vi "Main.vi"() -> ()   [LabVIEW 2021]
doc: "The myRIO Project template acquires acceleration data from the onboard accelerometer and displays the changes of acceleration values in a waveform chart."
uses:
  <vilib>/userDefined/High Color/IMAQdx.ctl
  <vilib>/vision/driver/IMAQdx.llb/IMAQdx Camera Control Mode.ctl
  <vilib>/vision/driver/IMAQdx.llb/IMAQdx Acquisition Mode.ctl
  <vilib>/vision/driver/IMAQdx.llb/IMAQdx Buffer Number Mode.ctl
  <vilib>/vision/Management.llb/Cast Image 2 Method.ctl
  <vilib>/Platform/TimedLoop/XDataNode/timing_clust.ctl
  <vilib>/Platform/TimedLoop/XDataNode/nitl_modes.ctl
  <vilib>/Platform/TimedLoop/XDataNode/wakeup.ctl
  <vilib>/myRIO/Instrument Drivers/Onboard IO/DIO/typedefs/DIO Reference.ctl
  <vilib>/myRIO/Common/Instrument Driver Framework/Utilities/typedefs/myRIO Generic Hardware Reference.ctl
  <vilib>/myRIO/Common/Instrument Driver Framework/Utilities/typedefs/Hardware Version Enum.ctl
  <vilib>/myRIO/Common/Instrument Driver Framework/Utilities/typedefs/myRIO v1.0 Reference.ctl
  <vilib>/myRIO/Common/Instrument Driver Framework/Utilities/typedefs/Generic FPGA Reference.ctl
  <vilib>/myRIO/Common/Instrument Driver Framework/myRIO v1.0/DIO/typedefs/DIO Channels List.ctl
  <vilib>/myRIO/Common/Instrument Driver Framework/myRIO v1.0/DIO/typedefs/DIO Channels Enum.ctl
  <vilib>/userDefined/High Color/nirio_resource_hc.ctl
  <vilib>/myRIO/Instrument Drivers/Onboard IO/AI/typedefs/AI Reference.ctl
  <vilib>/myRIO/Common/Instrument Driver Framework/myRIO v1.0/AI/typedefs/AI Channels List.ctl
  <vilib>/myRIO/Common/Instrument Driver Framework/myRIO v1.0/AI/typedefs/AI Channels Enum.ctl
  <vilib>/myRIO/Common/Instrument Driver Framework/Utilities/typedefs/Analog Scaling Constants List.ctl
  <vilib>/myRIO/Common/Instrument Driver Framework/Utilities/typedefs/Analog Scaling Constants.ctl
  <vilib>/myRIO/Instrument Drivers/Onboard IO/PWM/typedefs/PWM Reference.ctl
  <vilib>/myRIO/Common/Instrument Driver Framework/myRIO v1.0/PWM/typedefs/PWM Channels Enum.ctl
  <vilib>/myRIO/Instrument Drivers/Onboard IO/PWM/typedefs/PWM Configuration.ctl
  <vilib>/myRIO/Common/Instrument Driver Framework/myRIO v1.0/DIO/vis/myRIO v1.1 Open DIO.vi
  <vilib>/myRIO/Common/Instrument Driver Framework/myRIO v1.0/AI/vis/myRIO v1.1 Open AI.vi
  <vilib>/myRIO/Common/Instrument Driver Framework/Utilities/vis/Is FPGA Ref Available.vi
  <vilib>/myRIO/Common/Instrument Driver Framework/myRIO v1.0/PWM/vis/myRIO v1.1 Open PWM.vi
  <vilib>/myRIO/Common/Instrument Driver Framework/Utilities/vis/Validate Channels.vi
  <vilib>/myRIO/Common/Instrument Driver Framework/myRIO v1.0/DIO/vis/myRIO v1.0 Reserve DIO.vi
  <vilib>/myRIO/Common/Instrument Driver Framework/myRIO v1.0/AI/vis/myRIO v1.0 Reserve AI.vi
  <vilib>/myRIO/Common/Instrument Driver Framework/myRIO v1.0/DIO/vis/myRIO v1.0 Close DIO.vi
  <vilib>/myRIO/Common/Instrument Driver Framework/myRIO v1.0/AI/vis/myRIO v1.0 Close AI.vi
  <vilib>/myRIO/Common/Instrument Driver Framework/myRIO v1.0/PWM/vis/myRIO v1.0 Reserve PWM.vi
  <vilib>/myRIO/Instrument Drivers/Onboard IO/PWM/vis/Set Duty Cycle and Frequency.vi
  <vilib>/myRIO/Common/Instrument Driver Framework/myRIO v1.0/PWM/vis/myRIO v1.0 Close PWM.vi
  <vilib>/myRIO/Common/Instrument Driver Framework/myRIO v1.0/Resource Manager/vis/myRIO v1.0 Reserve Channel List.vi
  <vilib>/myRIO/Common/Instrument Driver Framework/myRIO v1.0/DIO/vis/myRIO v1.0 Build MUX Configuration DIO.vi
  <vilib>/myRIO/Common/Instrument Driver Framework/myRIO v1.0/AI/vis/myRIO v1.0 Build MUX Configuration AI.vi
  <vilib>/myRIO/Common/Instrument Driver Framework/myRIO v1.0/DIO/vis/myRIO v1.0 Unreserve DIO.vi
  <vilib>/myRIO/Common/Instrument Driver Framework/myRIO v1.0/AI/vis/myRIO v1.0 Unreserve AI.vi
  <vilib>/myRIO/Common/Instrument Driver Framework/myRIO v1.0/PWM/vis/myRIO v1.0 Build MUX Configuration PWM.vi
  <vilib>/myRIO/Common/Instrument Driver Framework/myRIO v1.0/PWM/vis/myRIO v1.0 Unreserve PWM.vi
  <vilib>/myRIO/Common/Instrument Driver Framework/myRIO v1.0/Resource Manager/vis/myRIO v1.0 Reserve Channel.vi
  <vilib>/myRIO/Common/Instrument Driver Framework/myRIO v1.0/Resource Manager/vis/myRIO v1.0 Unreserve Channel.vi
  <vilib>/myRIO/Common/Instrument Driver Framework/myRIO v1.0/Resource Manager/vis/myRIO v1.0 Create Configuration List.vi
  <vilib>/myRIO/Common/Instrument Driver Framework/myRIO v1.0/Resource Manager/vis/myRIO v1.0 Unreserve Channel List.vi
  <vilib>/myRIO/Common/Instrument Driver Framework/myRIO v1.0/Resource Manager/vis/myRIO v1.0 Build Mutex Name.vi
  <vilib>/Utility/VariantDataType/GetNumericInfo.vi
  <vilib>/Utility/error.llb/Error Cluster From Error Code.vi
  <vilib>/myRIO/Common/Instrument Driver Framework/myRIO v1.0/myRIO v1.1 Open.vi
  <vilib>/myRIO/Common/Instrument Driver Framework/Utilities/vis/IO Manager.vi
  <vilib>/myRIO/Common/Instrument Driver Framework/Utilities/vis/Configuration Manager.vi
  <vilib>/myRIO/Common/Instrument Driver Framework/myRIO v1.0/Resource Manager/vis/myRIO v1.0 Configure IO.vi
  <vilib>/myRIO/Common/Instrument Driver Framework/myRIO v1.0/myRIO v1.0 Close.vi
  <vilib>/myRIO/Common/Instrument Driver Framework/myRIO v1.0/PWM/vis/myRIO v1.0 Write PWM.vi
  <vilib>/myRIO/Common/Instrument Driver Framework/myRIO v1.0/AI/vis/myRIO v1.0 Get Scaling Constants AI.vi
  <vilib>/myRIO/Common/Instrument Driver Framework/myRIO v1.0/DIO/vis/myRIO v1.0 Write DIO.vi
  <vilib>/myRIO/Common/Instrument Driver Framework/myRIO v1.0/AI/vis/myRIO v1.0 Read AI.vi
  <vilib>/myRIO/Common/Instrument Driver Framework/myRIO v1.0/DIO/vis/myRIO v1.0 Shutdown DIO.vi
  <vilib>/myRIO/Common/Instrument Driver Framework/myRIO v1.0/DIO/vis/myRIO v1.0 Read DIO.vi
  <vilib>/myRIO/Common/Instrument Driver Framework/myRIO v1.0/PWM/vis/myRIO v1.0 Shutdown PWM.vi
  <vilib>/myRIO/Instrument Drivers/Onboard IO/PWM/vis/myRIO PWM Open.xnode
  <vilib>/myRIO/Instrument Drivers/Onboard IO/AI/vis/myRIO AI Open.xnode
  <vilib>/myRIO/Instrument Drivers/Onboard IO/DIO/vis/myRIO DIO Open.xnode
  <vilib>/platform/TimedLoop/XDataNode/XDataNode.xnode
  <vilib>/myRIO/Express VI/Onboard Devices/LED/LED Express VI.xnode
  <vilib>/vision/driver/NI_Vision_Acquisition_Software.lvlib
  <vilib>/vision/NI_Vision_Development_Module.lvlib
  <vilib>/myRIO/Instrument Drivers/Onboard IO/PWM/PWM.lvlib
  <vilib>/myRIO/Instrument Drivers/Onboard IO/DIO/DIO.lvlib
  <vilib>/myRIO/Instrument Drivers/Onboard IO/AI/AI.lvlib
  <vilib>/Platform/TimedLoop/XDataNode/XDNodeRunTimeDep.lvlib
panel:
  in  "error in (no error) 3":errorcluster
  out "Darkness level":dbl(slide) scale=0.0..1.0
  out "Numeric":dbl format="%.2f"
  in  "error in (no error) 2":errorcluster
  in  "error in (no error)":errorcluster
  out "error out 2":errorcluster
  out "error out":errorcluster
  in  "Stop":bool
  out "Image":T1(plugin-control)
  out "Is Colour from Sample Detected":bool
  out "Number of Circles Returned":i32
  out "Match Score":i32[](array[numeric])
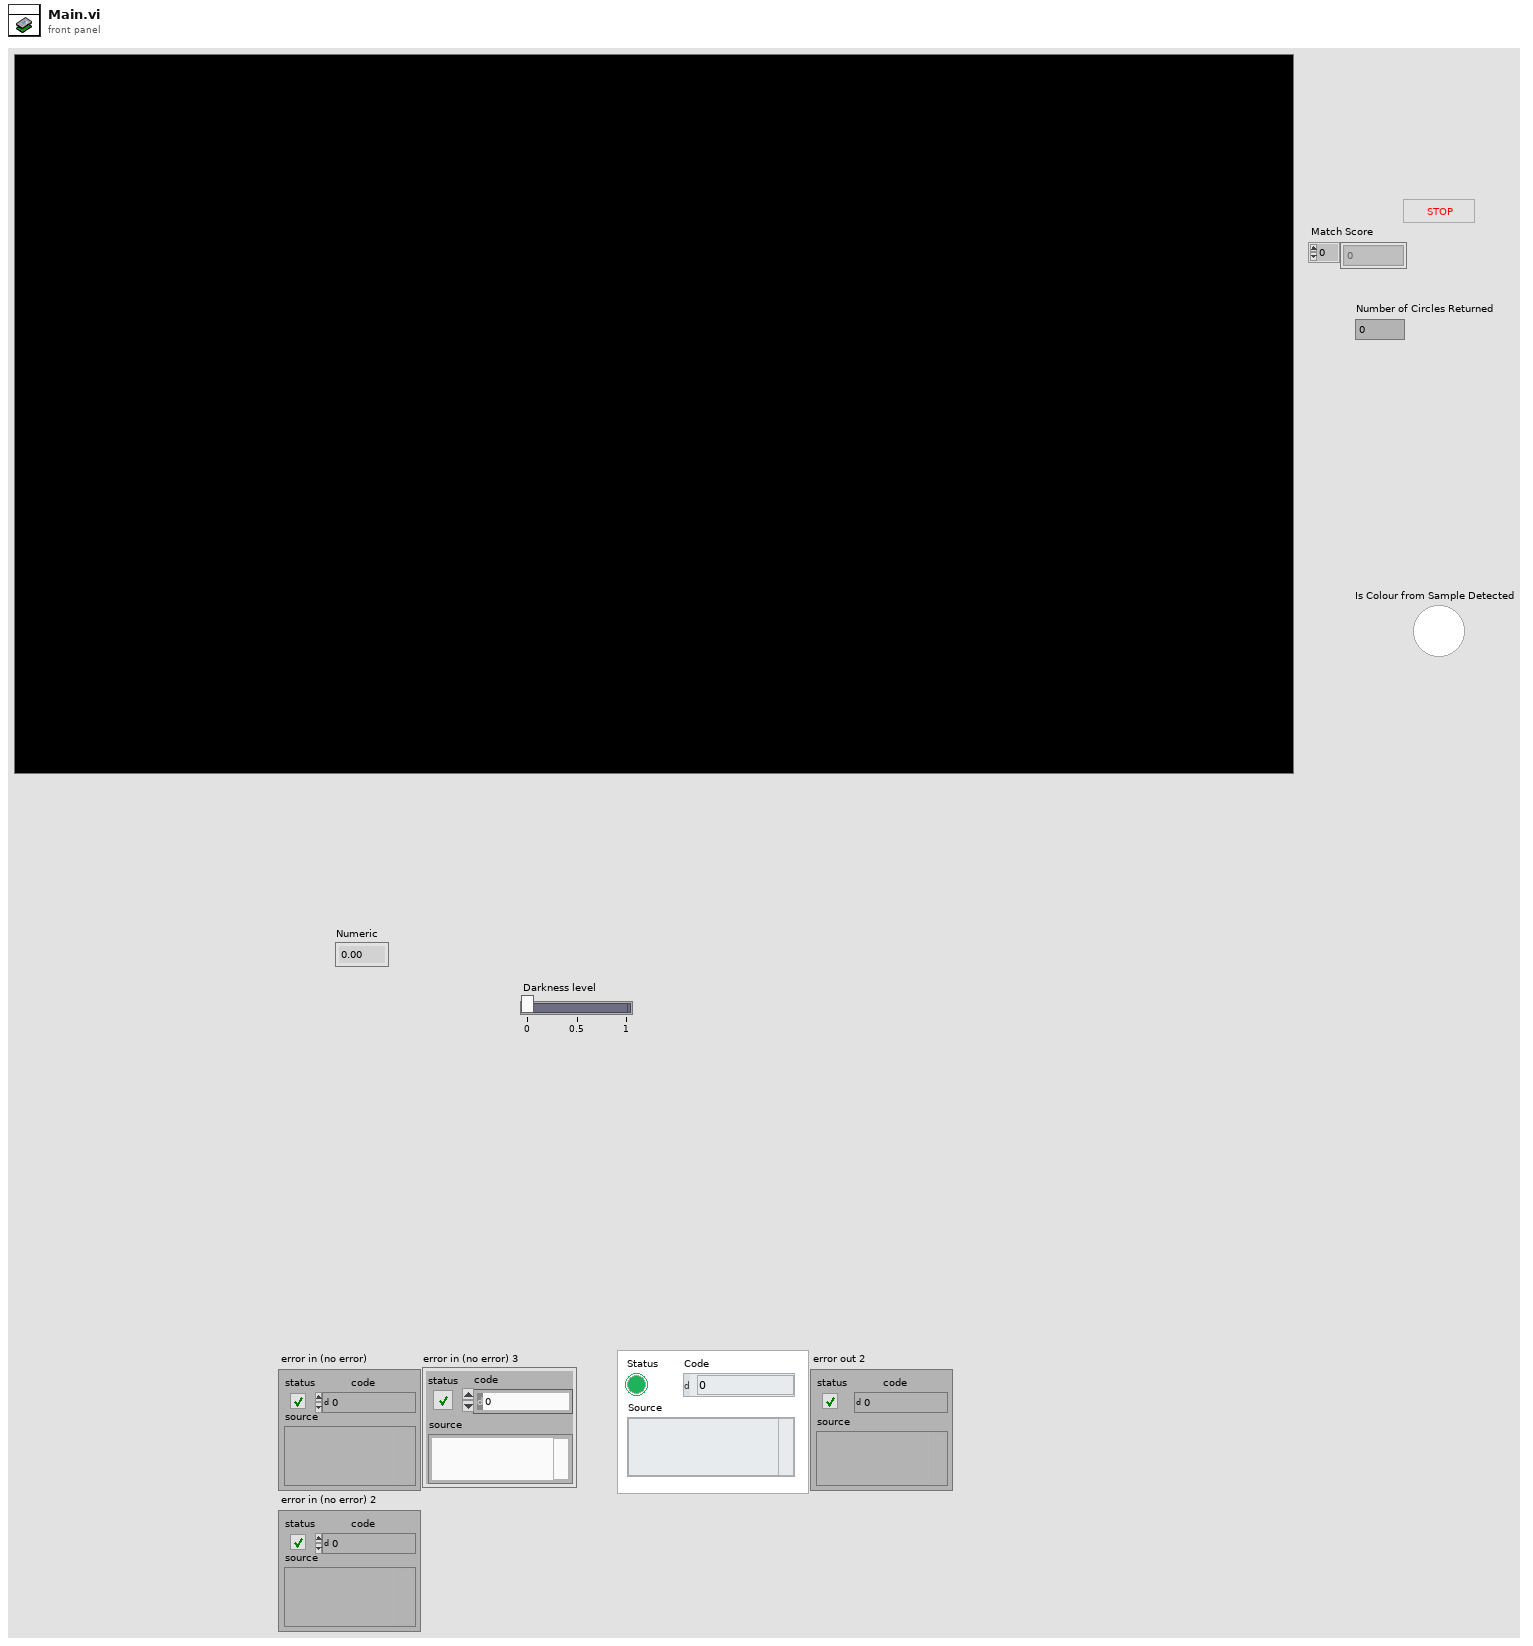
[diagram p1: front panel]
types:
  T1 = typedef "IMAQ Image.ctl" = refnum<image>
  T2 = typedef "Image Type" = u32
  T3 = typedef "Cast Image 2 Method.ctl" = u32
  T4 = typedef "IMAQ Rectangle" = cluster{"Left":i32, "Top":i32, "Right":i32, "Bottom":i32, "Rotation":dbl}
  T5 = typedef "NI_Vision_Acquisition_Software.lvlib/IMAQdx Buffer Number Mode.ctl" = enum32{"Next", "Last", "Buffer Number", "Every", "Last New"}
  T6 = typedef "NI_Vision_Acquisition_Software.lvlib/IMAQdx Acquisition Mode.ctl" = enum32{"One Shot", "Continuous"}
  T7 = typedef "NI_Vision_Acquisition_Software.lvlib/IMAQdx Camera Control Mode.ctl" = enum32{"Controller", "Listener"}
  T8 = typedef "IMAQdx.ctl" = refnum<k21>
  T9 = typedef "DIO.lvlib/DIO Reference.ctl" = cluster{"myRIO Reference":T10, "DIO Channels List":T14}
  T10 = typedef "myRIO Generic Hardware Reference.ctl" = cluster{"myRIO Model":T11, "myRIO Hardware Reference":T12}
  T11 = typedef "Hardware Version Enum.ctl" = enum16{"Unknown", "myRIO-1900", "myRIO-1950", "roboRIO", "NI ELVIS RIO CM", "ELVIS III"}
  T12 = typedef "myRIO v1.0 Reference.ctl" = cluster{"Generic FPGA Reference":T13, "Allow multiple opens":bool}
  T13 = typedef "Generic FPGA Reference.ctl" = refnum<k20>
  T14 = typedef "DIO Channels List.ctl" = T15[]
  T15 = typedef "DIO Channels Enum.ctl" = enum16{"Not Connected", "C/DIO0", "C/DIO1", "C/DIO2", "C/DIO3", "C/DIO4", "C/DIO5", "C/DIO6", "C/DIO7", "A/DIO0", "A/DIO1", "A/DIO2", "A/DIO3", "A/DIO4", "A/DIO5", "A/DIO6", "A/DIO7", "A/DIO8", "A/DIO9", "A/DIO10", "A/DIO11", "A/DIO12", "A/DIO13", "A/DIO14", "A/DIO15", "A/DIO16", "A/DIO17", "A/DIO18", "A/DIO19", "B/DIO0", "B/DIO1", "B/DIO2", "B/DIO3", "B/DIO4", "B/DIO5", "B/DIO6", "B/DIO7", "B/DIO8", "B/DIO9", "B/DIO10", "B/DIO11", "B/DIO12", "B/DIO13", "B/DIO14", "B/DIO15", "B/DIO16", "B/DIO17", "B/DIO18", "B/DIO19", "LED0", "LED1", "LED2", "LED3", "Button0", "DIO/DIO0", "DIO/DIO1", "DIO/DIO2", "DIO/DIO3", "DIO/DIO4", "DIO/DIO5", "DIO/DIO6", "DIO/DIO7", "DIO/DIO8", "DIO/DIO9", "SPI/CS0", "SPI/CS1", "SPI/CS2", "SPI/CS3", "LED RADIO (Green)", "LED RADIO (Red)", "LED COMM (Green)", "LED COMM (Red)", "LED MODE (Green)", "LED MODE (Red)"}
  T16 = typedef "XDNodeRunTimeDep.lvlib/timing_clust.ctl" = cluster{"Expected End [f-1]":u64, "Actual End [f-1]":u64, "Finished Late? [f-1]":bool, "Expected End [i-1]":u64, "Actual End [i-1]":u64, "Finished Late? [i-1]":bool, "Expected Start [i]":u64, "Actual Start [i]":u64, "Expected Start [f]":u64, "Actual Start [f]":u64, "Source Name":string, "Structure Name":string, "Period":i64, "Deadline":i64, "Offset":i64, "Start":i64, "Priority":i32, "Timeout":i32, "Mode":T17, "Wakeup Reason":T18, "Error":errorcluster, "Source Type":string, "Secondary Source Type":string, "Global End Time":u64, "Global Start Time":u64, "Frame Duration":u64, "Iteration Duration":u64, "Assigned CPU":i32, "I/O Scan Engine Mode":u32}
  T17 = typedef "XDNodeRunTimeDep.lvlib/nitl_modes.ctl" = enum32{"No Change", "Process missed periods, maintain original phase", "Discard missed periods, maintain original phase", "Process missed periods, ignore original phase", "Discard missed periods, ignore original phase"}
  T18 = typedef "XDNodeRunTimeDep.lvlib/wakeup.ctl" = enum32{"Normal", "Aborted", "Asynchronous wakeup", "Timing source error", "Timed loop error", "Timeout"}
  T19 = typedef "AI.lvlib/AI Reference.ctl" = cluster{"myRIO Reference":T10, "AI Channels List":T20, "AI Scaling Constants List":T22}
  T20 = typedef "AI Channels List.ctl" = T21[]
  T21 = typedef "AI Channels Enum.ctl" = enum16{"Not Connected", "AudioIn/Left", "AudioIn/Right", "C/AI0", "C/AI1", "A/AI0", "A/AI1", "A/AI2", "A/AI3", "A/AI4", "A/AI5", "A/AI6", "A/AI7", "B/AI0", "B/AI1", "B/AI2", "B/AI3", "B/AI4", "B/AI5", "B/AI6", "B/AI7", "AI/AI0", "AI/AI1", "AI/AI2", "AI/AI3", "A/AI0 (DIFF)", "A/AI1 (DIFF)", "A/AI2 (DIFF)", "A/AI3 (DIFF)", "B/AI0 (DIFF)", "B/AI1 (DIFF)", "B/AI2 (DIFF)", "B/AI3 (DIFF)"}
  T22 = typedef "Analog Scaling Constants List.ctl" = T23[]
  T23 = typedef "Analog Scaling Constants.ctl" = cluster{"LSB Weight (Volts)":dbl, "Offset (Volts)":dbl, "Signed?":bool}
  T24 = typedef "nirio_resource_hc.ctl" = tag
  T25 = typedef "PWM.lvlib/PWM Reference.ctl" = cluster{"myRIO Reference":T10, "PWM Channels Enum":T26, "PWM Configuration":T27}
  T26 = typedef "PWM Channels Enum.ctl" = enum16{"Not Connected", "C/PWM0", "C/PWM1", "A/PWM0", "A/PWM1", "A/PWM2", "A/PWM3", "A/PWM4", "A/PWM5", "A/PWM6", "A/PWM7", "A/PWM8", "A/PWM9", "A/PWM10", "A/PWM11", "A/PWM12", "A/PWM13", "A/PWM14", "A/PWM15", "A/PWM16", "A/PWM17", "A/PWM18", "A/PWM19", "B/PWM0", "B/PWM1", "B/PWM2", "B/PWM3", "B/PWM4", "B/PWM5", "B/PWM6", "B/PWM7", "B/PWM8", "B/PWM9", "B/PWM10", "B/PWM11", "B/PWM12", "B/PWM13", "B/PWM14", "B/PWM15", "B/PWM16", "B/PWM17", "B/PWM18", "B/PWM19", "PWM/PWM0", "PWM/PWM1", "PWM/PWM2", "PWM/PWM3", "PWM/PWM4", "PWM/PWM5", "PWM/PWM6", "PWM/PWM7", "PWM/PWM8", "PWM/PWM9"}
  T27 = typedef "PWM.lvlib/PWM Configuration.ctl" = cluster{"Frequency":dbl, "Duty Cycle":dbl}
  T28 = typedef "ROI Descriptor" = cluster{"Global Rectangle":i32[], "Contours":cluster{"ID":enum32{"External", "Internal"}, "Type":u32, "Coordinates":i32[]}[]}
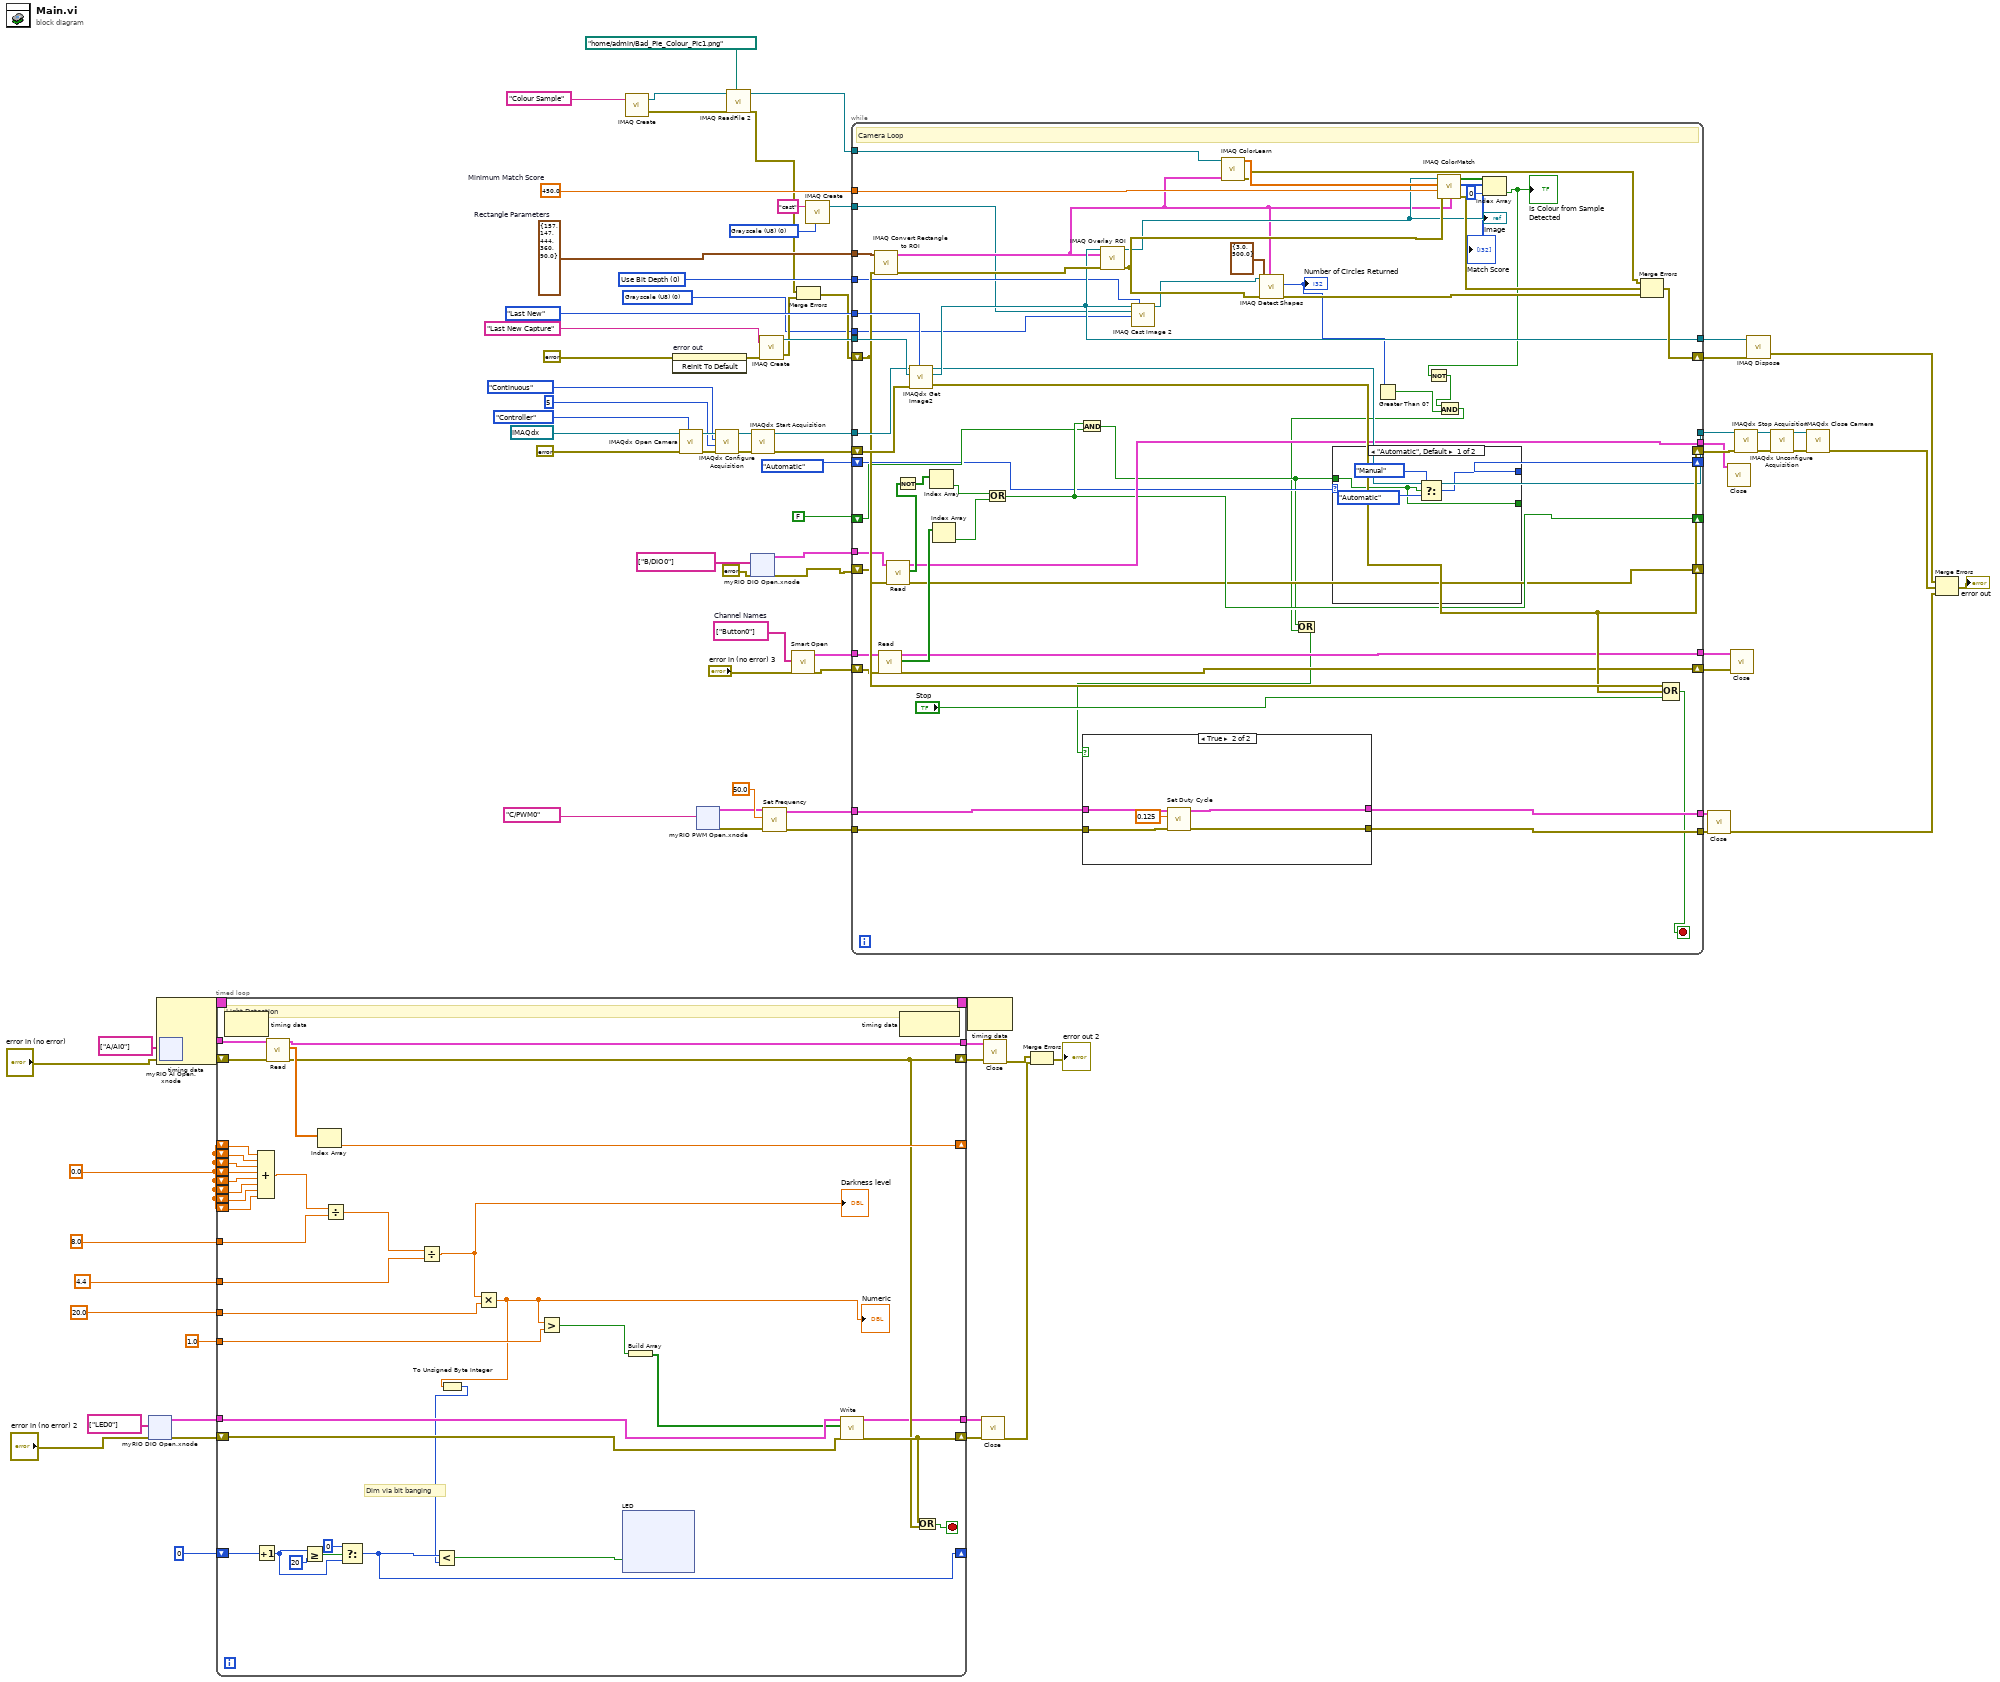
[diagram p0: block diagram]
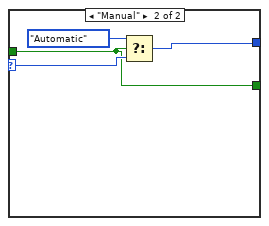
[diagram p2: hidden frame]
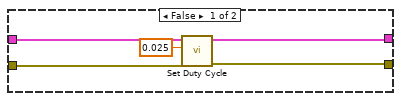
[diagram p3: hidden frame]
diagram:
  w12 = tag[] ["Button0"]  # Channel Names
  w30 = 0.0
  w36 = T2 0 items=["Grayscale (U8)", "Grayscale (I16)", "Grayscale (SGL)", "Complex (CSG)", "RGB (U32)", "HSL (U32)", "RGB (U64)", "Grayscale (U16)"] ("Image Type")
  w42 = T3 0 items=["Use Bit Depth", "Shift", "Use Lookup Table"] ("Method")
  w43 = T2 0 items=["Grayscale (U8)", "Grayscale (I16)", "Grayscale (SGL)", "Complex (CSG)", "RGB (U32)", "HSL (U32)", "RGB (U64)", "Grayscale (U16)"] ("Image Type")
  w53 = 450.0  # Minimum Match Score
  w60 = T4 {"Left"=157, "Top"=147, "Right"=444, "Bottom"=360, "Rotation"=90.0}  # Rectangle Parameters
  n1 = xnode "myRIO DIO Open.xnode"("error in (no error)"="error in (no error) 2", "Channel Names"=tag[] ["LED0"]) -> ("error out"=w25:errorcluster, "DIO Ref Out"=w26:T9)  [unwired: 1 in]
  n2 = node-c288() -> (w87:T16)  [unwired: 4 in]
  n3 = xnode "myRIO AI Open.xnode"("error in (no error)"="error in (no error)", "Channel Names"=tag[] ["A/AI0"]) -> ("error out"=w33:errorcluster, "AI Ref Out"=w34:T19)  [unwired: 1 in]
  n4 = timed-loop {
    tunnel: w34 -> [w124]
    shift-right: [w102] -> w32
    shift-left: w33 -> [w123]
    tunnel: [w122] -> w31
    shift-right: [w112] -> _
    shift-left: w30 -> [w114]
    shift-left: w30 -> [w115]
    shift-left: w30 -> [w116]
    shift-left: w30 -> [w117]
    shift-left: w30 -> [w118]
    shift-left: w30 -> [w119]
    shift-left: w30 -> [w120]
    shift-left: w30 -> [w121]
    tunnel: 8.0 -> [w111]
    tunnel: 4.4 -> [w109]
    tunnel: 20.0 -> [w107]
    tunnel: w26 -> [w105]
    shift-right: [w103] -> w24
    shift-left: w25 -> [w104]
    tunnel: [w101] -> w23
    tunnel: 1.0 ("y") -> [w99]
    shift-right: [w91] -> _
    shift-left: u8 0 -> [w93]
    timing: w87 -> [_]
    timing-out: [_] -> w86
    stop <- w100 stop-if-true
    # "Dim via bit banging"
    # "Light Detection"
    n5 = node-c288() -> ()  [unwired: 1 in, 1 out]
    n6 = Increment(x=w93) -> (x+1=w88:u8)
    n7 = Compound Arithmetic op=ADD(w114, w115, w116, w117, w118, w119, w120, w121) -> (w110:dbl)
    n8 = call <vilib>:"Read.vi"("error in (no error)"=w123, "AI Ref In"=w124) -> ("error out"=w102:errorcluster, "Values"=w113:dbl[], "AI Ref Out"=w122:T19)  [unwired: 7 in]
    n9 = Greater Or Equal?(x=w88, y=u8 20) -> (x >= y?=w95:bool)
    n10 = Index Array(array=w113) -> (element=w112:dbl)  [unwired: 1 in]
    n11 = Divide(x=w110, y=w111) -> (x/y=w108:dbl)
    n12 = Select(t=u8 0, s=w95, f=w88) -> (s? t:f=w91:u8)
    n13 = Divide(x=w108, y=w109) -> (x/y=w106:dbl)
    "Darkness level" <- w106
    n14 = Multiply(x=w106, y=w107) -> (x*y=w90:dbl)
    "Numeric" <- w90
    n15 = To Unsigned Byte Integer(number=w90) -> (unsigned 8bit integer=w89:u8)
    n16 = Less?(x=w91, y=w89) -> (x < y?=w92:bool)
    n17 = Greater?(x=w90, y=w99) -> (0:w98:bool)
    n18 = xnode "LED"("LED Activation"=w92) -> ()  [unwired: 1 in, 1 out]
    n19 = Build Array(w98) -> (w97:bool[])
    n20 = call <vilib>:"Write.vi"("error in (no error)"=w104, "Values"=w97, "DIO Ref In"=w105) -> ("error out"=w103:errorcluster, "DIO Ref Out"=w101:T9)  [unwired: 6 in]
    n21 = node-c288() -> ()  [unwired: 1 in, 1 out]
    n22 = Or(x=w103, y=w102) -> (x .or. y?=w100:bool)
  }
  n23 = call "IMAQ Create"("Image Name"="Colour Sample") -> ("New Image"=w56:T1, "error out"=w54:errorcluster)  [unwired: 4 in]
  n24 = invoke on="error out" class="Clust (strict)" method="Reinit To Default"(error in=errorcluster {"status"=FALSE, "code"=0, "source"=""}) -> (error out=w62:errorcluster)  [unwired: 2 in, 2 out]
  n25 = call <vilib>:"IMAQdx Open Camera.vi"("Camera Control Mode"=IMAQdx_Camera_Control_Mode."Controller", "error in"=errorcluster {"status"=FALSE, "code"=0, "source"=""}, "Session In"=T8 "cam0") -> ("error out"=w85:errorcluster, "Session Out"=w84:T8)  [unwired: 7 in]
  n26 = xnode "myRIO PWM Open.xnode"("Channel Name"=tag "C/PWM0") -> ("error out"=w48:errorcluster, "PWM Ref Out"=w50:T25)  [unwired: 2 in]
  n27 = call <vilib>:"IMAQdx Configure Acquisition.vi"("error in"=w85, "Number of Buffers"=u32 5, "Continuous?"=IMAQdx_Acquisition_Mode."Continuous", "Session In"=w84) -> ("error out"=w79:errorcluster, "Session Out"=w78:T8)  [unwired: 6 in]
  n28 = call "IMAQ ReadFile 2"("File Path"=path "/home/admin/Bad_Pie_Colour_Pic1.png", "error in (no error)"=w54, "Image"=w56) -> ("error out"=w41:errorcluster, "Image Out"=w55:T1)  [unwired: 4 in, 3 out]
  n29 = xnode ("myRIO DIO Open.xnode")("error in (no error)"=errorcluster {"status"=FALSE, "code"=0, "source"=""}, "Channel Names"=tag[] ["B/DIO0"]) -> ("error out"=w7:errorcluster, "DIO Ref Out"=w4:T9)  [unwired: 1 in]
  n30 = call <vilib>:"IMAQdx Start Acquisition.vi"("error in"=w79, "Session In"=w78) -> ("error out"=w72:errorcluster, "Session Out"=w70:T8)  [unwired: 8 in]
  n31 = call "IMAQ Create"("Image Name"="Last New Capture", "error in (no error)"=w62) -> ("New Image"=w67:T1, "error out"=w44:errorcluster)  [unwired: 3 in]
  n32 = call <vilib>:"Set Frequency.vi"("error in (no error)"=w48, "Frequency [Hz]"=50.0, "PWM Ref In"=w50) -> ("error out"=w47:errorcluster, "PWM Ref Out"=w49:T25)  [unwired: 6 in]
  n33 = call <vilib>:"Smart Open.vi"("error in (no error)"="error in (no error) 3", "Channel Names"=w12) -> ("error out"=w6:errorcluster, "DIO Ref Out"=w5:T9)  [unwired: 8 in]
  n34 = Merge Errors(w41, w44) -> (w58:errorcluster)
  n35 = call "IMAQ Create"("Image Name"="cast", "Image Type"=w36) -> ("New Image"=w35:T1)  [unwired: 3 in, 1 out]
  n36 = while {
    shift-right: [w197] -> w71
    shift-left: w72 -> [w215]
    tunnel: w70 -> [w216]
    tunnel: [w196] -> w69
    tunnel: IMAQdx_Buffer_Number_Mode."Last New" ("Buffer Number Mode (Next)") -> [w219]
    shift-right: [w207] -> w64
    shift-left: w58 -> [w211]
    tunnel: w67 -> [w218]
    tunnel: [w201] -> w65
    tunnel: w60 -> [w214]
    tunnel: w55 -> [w195]
    tunnel: w53 -> [w206]
    tunnel: w49 -> [w194]
    tunnel: w47 -> [w192]
    tunnel: [w193] -> w46
    tunnel: [w191] -> w45
    tunnel: w43 -> [w199]
    tunnel: w42 -> [w198]
    tunnel: w35 -> [w187]
    shift-right: [w171] -> _
    shift-left: enum16{"Automatic", "Manual"}."Automatic" -> [w165]
    shift-right: [w170] -> _
    shift-left: FALSE -> [w166]
    shift-right: [w167] -> _
    shift-left: w7 -> [w175]
    shift-right: [w169] -> w2
    shift-left: w6 -> [w173]
    tunnel: w5 -> [w174]
    tunnel: w4 -> [w176]
    tunnel: [w172] -> w3
    tunnel: [w168] -> w1
    stop <- w190 stop-if-true
    # "Camera Loop"
    n37 = call "IMAQ Convert Rectangle to ROI"("error in (no error)"=w211, "Rectangle"=w214) -> ("error out"=w213:errorcluster, "ROI Descriptor"=w188:T28)  [unwired: 7 in]
    n38 = call <vilib>:"Read.vi"("error in (no error)"=w173, "DIO Ref In"=w174) -> ("error out"=w169:errorcluster, "Values"=w181:bool[], "DIO Ref Out"=w168:T9)  [unwired: 7 in]
    n39 = call <vilib>:"Read.vi"("error in (no error)"=w175, "DIO Ref In"=w176) -> ("error out"=w167:errorcluster, "Values"=w179:bool[], "DIO Ref Out"=w172:T9)  [unwired: 7 in]
    n40 = Not(x=w179) -> (.not. x?=w180:bool[])
    n41 = call <vilib>:"IMAQdx Get Image2.vi"("Buffer Number Mode (Next)"=w219, "error in"=w215, "Image In"=w218, "Session In"=w216) -> ("error out"=w197:errorcluster, "Image Out"=w201:T1, "Session Out"=w196:T8)  [unwired: 4 in, 1 out]
    n42 = Index Array "Index Array"(array=w180) -> (element=w177:bool)  [unwired: 1 in]
    n43 = Index Array(array=w181) -> (element=w178:bool)  [unwired: 1 in]
    n44 = Or(x=w177, y=w178) -> (x .or. y?=w170:bool)
    n45 = And(x=w170, y=w166) -> (x .and. y?=w164:bool)
    n46 = call "IMAQ Overlay ROI"("error in (no error)"=w213, "ROI Descriptor"=w188, "Image"=w201) -> ("error out"=w205:errorcluster, "Image Out"=w202:T1)  [unwired: 7 in]
    "Image" <- w202
    n47 = call "IMAQ Cast Image 2"("Image Src"=w201, "Method"=w198, "Image Dst"=w187, "Image Type"=w199) -> ("Image Dst Out"=w200:T1)  [unwired: 10 in, 1 out]
    n48 = call "IMAQ ColorLearn"("ROI Descriptor"=w188, "Image"=w195) -> ("Color Spectrum"=w212:dbl[], "error out"=w189:errorcluster)  [unwired: 6 in]
    n49 = call-poly "IMAQ Detect Shapes"("ROI Descriptor"=w188, "error in (no error)"=w205, "Circle Descriptor"=cluster{"Min Radius":dbl, "Max Radius":dbl} {"Min Radius"=3.0, "Max Radius"=500.0}, "Image"=w200) -> ("error out"=w204:errorcluster, "Number of Matches Returned"=w185:i32)  [unwired: 5 in, 1 out]
    "Number of Circles Returned" <- w185
    n50 = case shown="\"Automatic\", Default" w165 {
      selector: w165 -> [_ w225]
      tunnel: [w223 w226] -> w171
      tunnel: w164 -> [w220 w224]
      tunnel: [w220 w224] -> _
      frame "Automatic", Default {
        n51 = Select(t=enum16{"Automatic", "Manual"}."Manual", s=w220, f=enum16{"Automatic", "Manual"}."Automatic") -> (s? t:f=w223:enum16{"Automatic", "Manual"})
      }
      frame "Manual" {
        n52 = Select(t=enum16{"Automatic", "Manual"}."Automatic", s=w224, f=w225) -> (s? t:f=w226:enum16{"Automatic", "Manual"})
      }
    }
    n53 = Greater Than 0?(x=w185) -> (x > 0?=w184:bool)
    n54 = call "IMAQ ColorMatch"("ROI Descriptor"=w188, "Image"=w202, "Color Spectrum"=w212, "Minimum Match Score"=w206, "error in (no error)"=w205) -> ("Match Flag"=w210:bool[], "Match Score"=→"Match Score":i32[], "error out"=w208:errorcluster)  [unwired: 2 in]
    n55 = Index Array "Index Array"(array=w210, index=0) -> (element=w182:bool)
    "Is Colour from Sample Detected" <- w182
    n56 = Not(x=w182) -> (.not. x?=w183:bool)
    n57 = And(x=w183, y=w184) -> (x .and. y?=w163:bool)
    n58 = Or(x=w164, y=w163) -> (x .or. y?=w162:bool)
    n59 = case shown="True" w162 {
      tunnel: w194 -> [w232 w237]
      tunnel: [w230 w236] -> w193
      tunnel: w192 -> [w231 w235]
      tunnel: [w229 w234] -> w191
      frame False {
        n60 = call <vilib>:"Set Duty Cycle.vi"("error in (no error)"=w231, "Duty Cycle"=0.025, "PWM Ref In"=w232) -> ("error out"=w229:errorcluster, "PWM Ref Out"=w230:T25)  [unwired: 6 in]
      }
      frame True {
        n61 = call <vilib>:"Set Duty Cycle.vi"("error in (no error)"=w235, "Duty Cycle"=0.125, "PWM Ref In"=w237) -> ("error out"=w234:errorcluster, "PWM Ref Out"=w236:T25)  [unwired: 6 in]
      }
    }
    n62 = Merge Errors(w189, w208, w204) -> (w207:errorcluster)
    n63 = Compound Arithmetic op=OR(w211, w197, "Stop") -> (w190:bool)
  }
  n64 = node-c288(w86) -> ()  [unwired: 1 out]
  n65 = call <vilib>:"Close.vi"("error in (no error)"=w24, "DIO Ref In"=w23) -> ("error out"=w20:errorcluster)  [unwired: 9 in]
  n66 = call <vilib>:"Close.vi"("error in (no error)"=w32, "AI Ref In"=w31) -> ("error out"=w21:errorcluster)  [unwired: 9 in]
  n67 = Merge Errors(w21, w20) -> (→"error out 2":errorcluster)
  n68 = call <vilib>:"Close.vi"("error in (no error)"=w45, "PWM Ref In"=w46) -> ("error out"=w38:errorcluster)  [unwired: 9 in]
  n69 = call <vilib>:"Close.vi"("DIO Ref In"=w3) -> ()  [unwired: 10 in, 1 out]
  n70 = call <vilib>:"Close.vi"("error in (no error)"=w2, "DIO Ref In"=w1) -> ()  [unwired: 9 in, 1 out]
  n71 = call <vilib>:"IMAQdx Stop Acquisition.vi"("error in"=w71, "Session In"=w69) -> ("error out"=w81:errorcluster, "Session Out"=w80:T8)  [unwired: 8 in]
  n72 = call "IMAQ Dispose"("Image"=w65, "error in (no error)"=w64) -> ("error out"=w40:errorcluster)  [unwired: 4 in]
  n73 = call <vilib>:"IMAQdx Unconfigure Acquisition.vi"("error in"=w81, "Session In"=w80) -> ("error out"=w83:errorcluster, "Session Out"=w82:T8)  [unwired: 8 in]
  n74 = call <vilib>:"IMAQdx Close Camera.vi"("error in"=w83, "Session In"=w82) -> ("error out"=w39:errorcluster)  [unwired: 9 in]
  n75 = Merge Errors(w40, w39, w38) -> (→"error out":errorcluster)
